vi "test_cmd.vi"() -> ()   [LabVIEW 2011]
panel:
  out "error out":errorcluster
  out "standard error":string
  out "standard output":string
  in  "Command":string
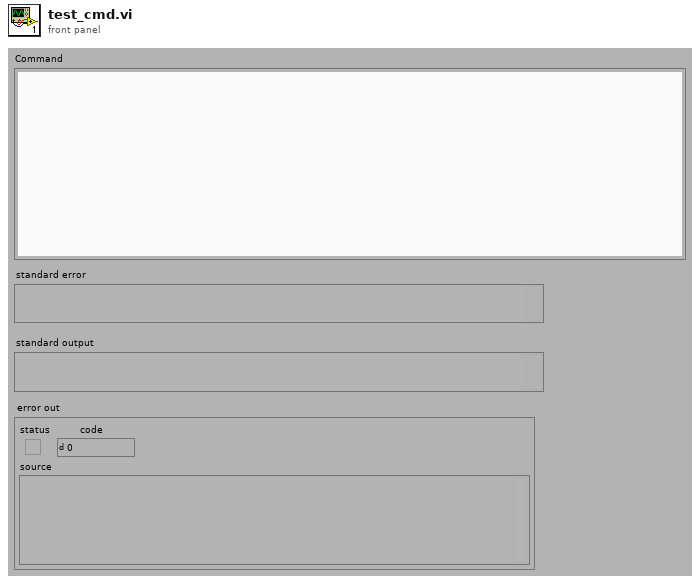
[diagram p1: front panel]
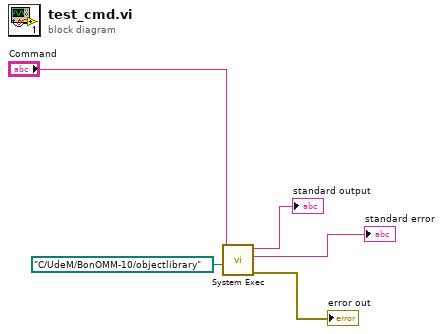
[diagram p0: block diagram]
diagram:
  n1 = call <vilib>:"System Exec.vi"("working directory"=path "C:/UdeM/BonOMM-10/objectlibrary", "command line"="Command") -> ("error out"=→"error out":errorcluster, "standard error"=→"standard error":string, "standard output"=→"standard output":string)  [unwired: 6 in, 1 out]
